vi "FRCts20_Backend_Test_Request_RawPostSpeed.vi"() -> ()   [LabVIEW 2014, in "FRCts20_Backend_TestCode.lvlib"]
uses:
  FRCts20_Backend_TestCode.lvlib
  <vilib>/addons/database/Connection.llb/DB Tools Open Connec (String).vi
  <vilib>/addons/database/NI_Database_API.lvlib
  FRCts20_Backend_Engine.lvlib
panel:
  out "rows affected":i32
  out "x-y":u32
  out "error out":errorcluster
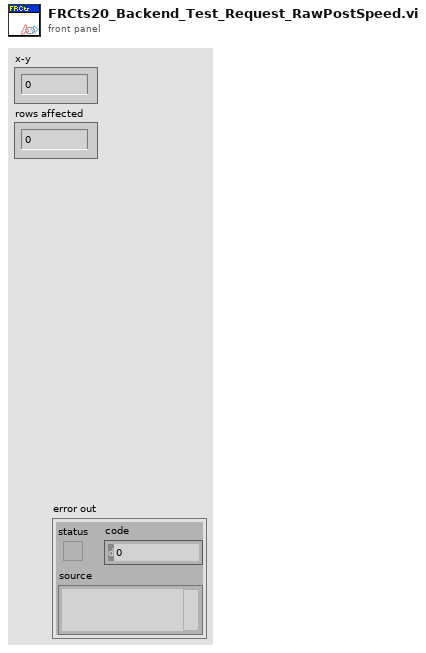
[diagram p1: front panel]
types:
  T1 = typedef "NI_Database_API.lvlib/Conn ObjectReference.ctl" = refnum<k1>
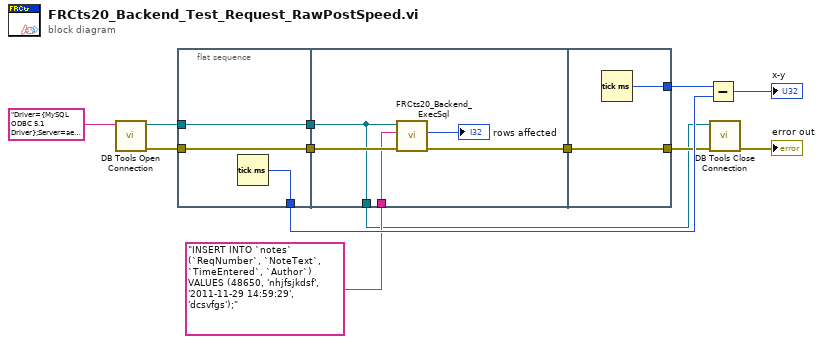
[diagram p0: block diagram]
diagram:
  n1 = call-poly <vilib>:"DB Tools Open Connection.vi"("connection information"="Driver={MySQL ODBC 5.1 Driver};Server=ae-assigner;Database=parkway;User=root; Password=password;Option=3;") -> ("error out"=w11:errorcluster, "connection reference"=w12:T1)  [unwired: 7 in]
  n2 = flat-sequence {
    tunnel: w11 -> [w15]
    tunnel: w12 -> [w16]
    tunnel: [w16] -> w10
    tunnel: [w15] -> w9
    tunnel: [w14] -> w6
    tunnel: w10 -> [w17]
    tunnel: w9 -> [w21]
    tunnel: [w20] -> w8
    tunnel: "INSERT INTO `notes` (`ReqNumber`, `NoteText`, `TimeEntered`, `Author`) VALUES (48650, 'nhjfsjkdsf', '2011-11-29 14:59:29', 'dcsvfgs');" -> [w19]
    tunnel: [w17] -> w1
    tunnel: [w23] -> w3
    tunnel: w8 -> [w23]
    tunnel: [w22] -> w7
    frame #0 {
      n3 = Tick Count (ms)() -> (millisecond timer value=w14:u32)
    }
    frame #1 {
      n4 = call "FRCts20_Backend_ExecSql.vi"("error in (no error)"=w21, "format string"=w19, "Refnum in"=w17) -> ("error out"=w20:errorcluster, "rows affected"=→"rows affected":i32)  [unwired: 6 in, 1 out]
    }
    frame #2 {
      n5 = Tick Count (ms)() -> (millisecond timer value=w22:u32)
    }
  }
  n6 = Subtract(x=w7, y=w6) -> (x-y=→"x-y":u32)
  n7 = call <vilib>:"DB Tools Close Connection.vi"("error in (no error)"=w3, "connection reference"=w1) -> ("error out"=→"error out":errorcluster)  [unwired: 5 in]
